vi "Periodic Tasks.vi"(8 "error in":errorcluster) -> ()   [LabVIEW 2016]
doc: "This VI runs in parallel to other tasks. It can contain as many user-defined periodic loops as you need. These can carry out PID or other sorts of timed response."
uses:
  <vilib>/Rock Robotics/WPI/Solenoid/WPI_SolenoidValue.ctl
  <vilib>/Rock Robotics/WPI/DriverStation/WPI_DriverStationRobotMode2.ctl
  <vilib>/Rock Robotics/WPI/Utilities/WPI_GetSetVariantRefNum.vi
  Robot Global Data.vi
  <vilib>/Rock Robotics/WPI/Solenoid/WPI_SolenoidSetEnum.vi
  Added Files/Apple Gyro/Apple Pi Gyro Library.lvlib
panel:
  out "Robot Centric?":bool
  in  "Turn":dbl=0.7 format="%#_13g"
  in  "Harvest Spd":dbl=0.9 format="%#_13g"
  out "Output":bool
  out "Intake":bool
  in  "Output":i32=6
  in  "Intake":i32=4
  out "Gyro Yaw Out 2":dbl format="%#_13g"
  in  "Rot Pt Y":dbl format="%#_13g"
  in  "Rot Pt X":dbl format="%#_13g"
  in  "Robot Centric":i32
  in  "Field Centric":i32
  in  "Y Axis":i32=1
  in  "Drive wait":u32=25
  out "Drive Loop Speed":u32=245
  in  "Slow Drive Speed %":dbl=0.65
  in  "OP wait":u32=25
  out "Op Loop Speed":u32=138
  out "Joystick Loop Speed":u32=39
  in  "Joystick wait":u32=25
  out "Reset Offsets":bool
  out "Vision Lineup":bool
  out "Driver 2 POV":i16=-1
  out "Climb":bool
  in  "Reset Offsets":i32=7
  in  "Lineup":i32
  in  "Drive Slow":i32=1
  in  "Gyro Reset":i32=2
  in  "Climb":i32=1
  in  "Max Climb Speed":dbl=-1.0
  # "Left Driver 1"
  # "Right Driver 2"
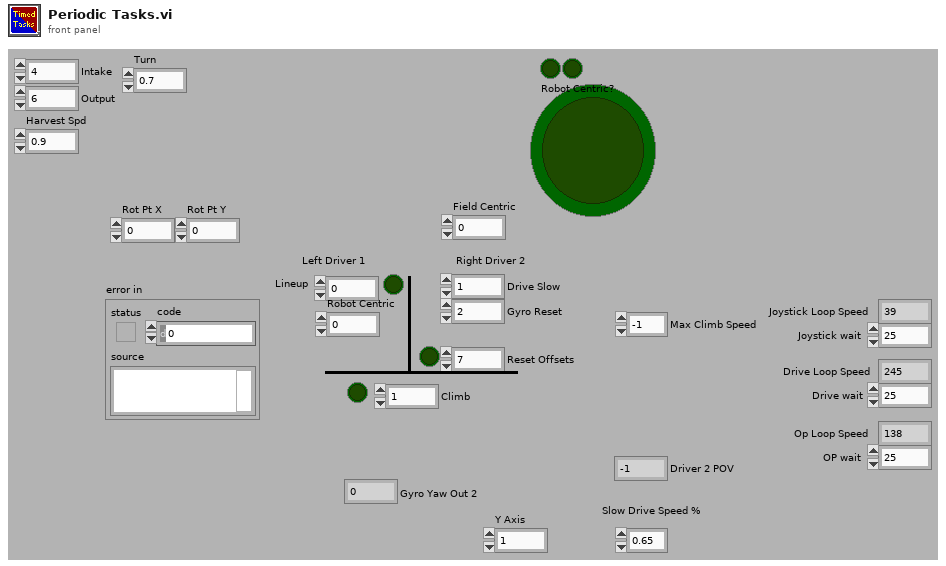
[diagram p1: front panel]
types:
  T1 = typedef "WPI_JoystickDevRef.ctl" = cluster{"Device":T2}
  T2 = typedef "WPI_JoystickDeviceEnum.ctl" = enum16{"USB 0", "USB 1", "USB 2", "USB 3", "USB 4", "USB 5"}
  T3 = typedef "WPI_DriverStationRobotMode2.ctl" = enum16{"Autonomous Disabled", "Autonomous Enabled", "Teleop Disabled", "Teleop Enabled", "Disconnected", "Finish", "Test Disabled", "Test Enabled", "Emergency Stopped"}
  T4 = typedef "WPI_MotorControlDeviceRef.ctl" = cluster{"DeviceStatus":errorcluster, "Type":T5, "PWM":cluster{"PWM Channel":T6, "DeadBand":T7}, "CAN":cluster{"Device Number":u8, "SetOutput VI Ref":variant, "GetOutput VI Ref":variant, "Enable VI Ref":variant, "Disable VI Ref":variant, "Data":variant}, "Invert":bool}
  T5 = typedef "WPI_MotorControlType.ctl" = enum16{"PWM", "CAN"}
  T6 = typedef "FPGA_DIOPWMChannel.ctl" = enum8{"PWM 0", "PWM 1", "PWM 2", "PWM 3", "PWM 4", "PWM 5", "PWM 6", "PWM 7", "PWM 8", "PWM 9", "PWM MXP 0", "PWM MXP 1", "PWM MXP 2", "PWM MXP 3", "PWM MXP 4", "PWM MXP 5", "PWM MXP 6", "PWM MXP 7", "PWM MXP 8", "PWM MXP 9", "Invalid"}
  T7 = typedef "WPI_PWMDeadband.ctl" = cluster{"Name":string, "maxPositivePwm":i32, "minPositivePwm":i32, "centerPwm":i32, "maxNegativePwm":i32, "minNegativePwm":i32, "angularRange":u16}
  T8 = typedef "WPI_SolenoidDevRef.ctl" = cluster{"DevStatus":errorcluster, "Pneumatics Control Module":u8, "Forward Solenoid Channel":T9, "Reverse Solenoid Channel":T9}
  T9 = typedef "WPI_SolenoidChannel.ctl" = enum8{"Solenoid 0", "Solenoid 1", "Solenoid 2", "Solenoid 3", "Solenoid 4", "Solenoid 5", "Solenoid 6", "Solenoid 7", "Invalid"}
  T10 = typedef "WPI_SolenoidValue.ctl" = enum16{"Off", "On", "Forward", "Reverse"}
  T11 = typedef "WPI_CompressorDevRef.ctl" = cluster{"DevStatus":errorcluster, "Pneumatics Control Module":u8}
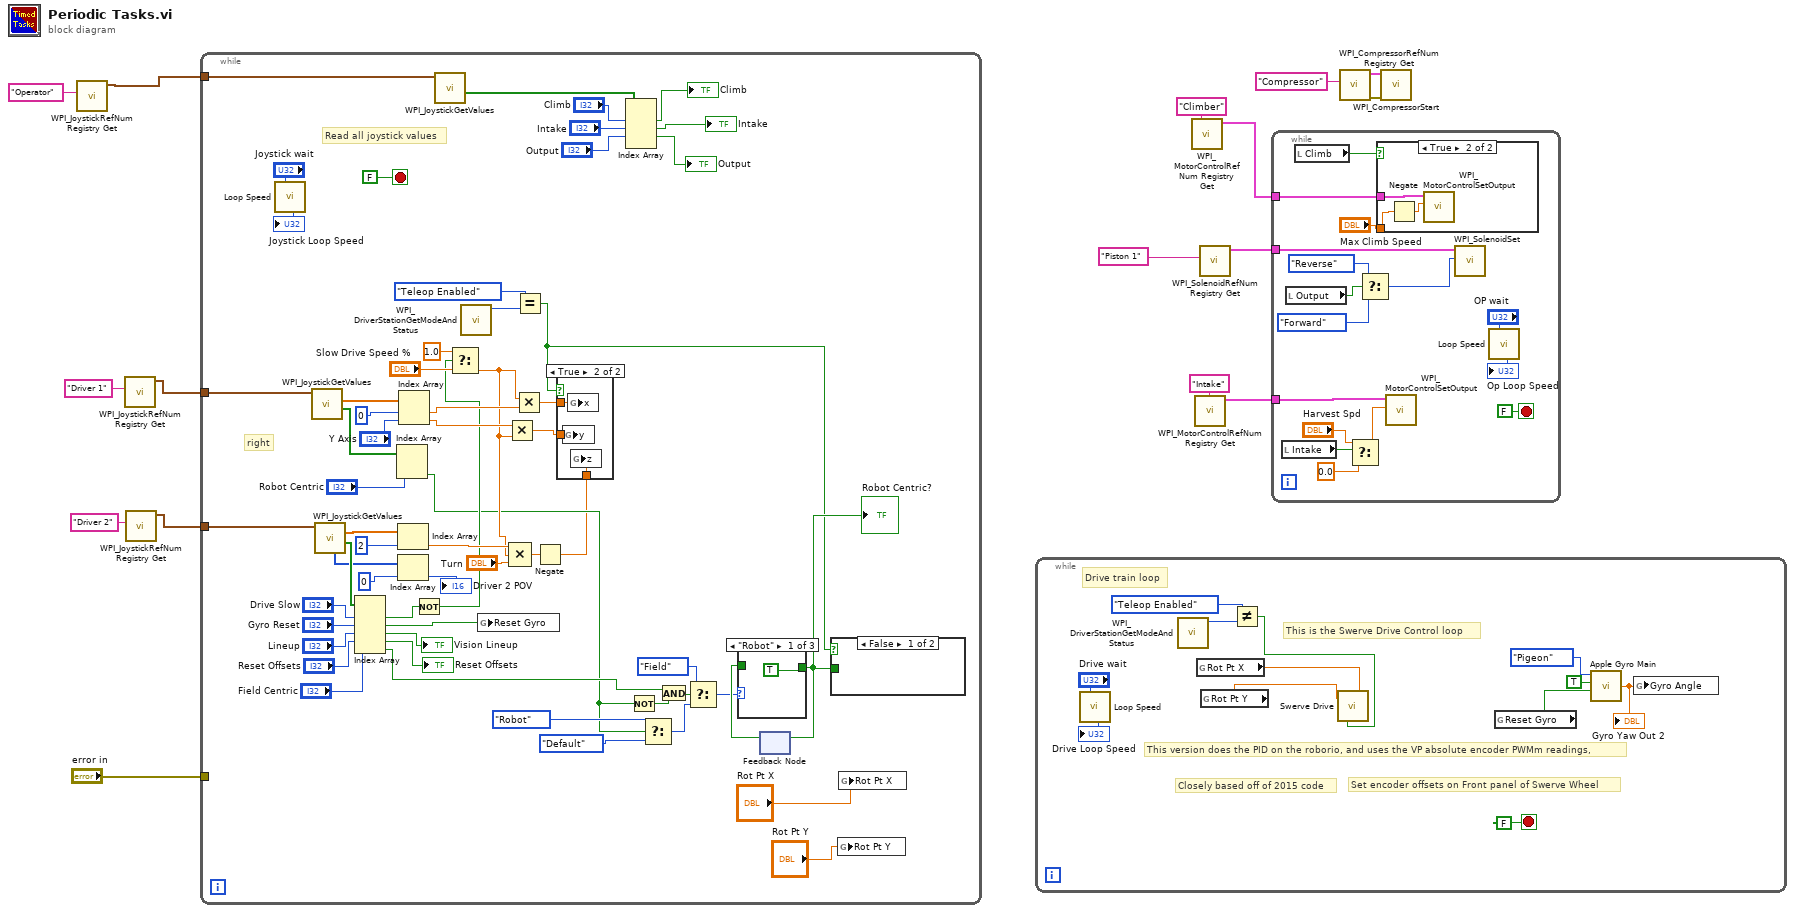
[diagram p0: block diagram]
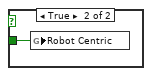
[diagram p2: hidden frame]
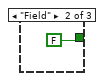
[diagram p4: hidden frame]
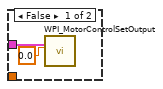
[diagram p6: hidden frame]
diagram:
  n1 = call <vilib>:"WPI_JoystickRefNum Registry Get.vi"("refnum name"="Operator") -> ("JoystickDevRef"=w11:T1)  [unwired: 9 in, 1 out]
  n2 = call <vilib>:"WPI_JoystickRefNum Registry Get.vi"("refnum name"="Driver 1") -> ("JoystickDevRef"=w10:T1)  [unwired: 9 in, 1 out]
  n3 = call <vilib>:"WPI_JoystickRefNum Registry Get.vi"("refnum name"="Driver 2") -> ("JoystickDevRef"=w9:T1)  [unwired: 9 in, 1 out]
  n4 = while {
    tunnel: w11 -> [w45]
    tunnel: w10 -> [w44]
    tunnel: w9 -> [w43]
    tunnel: "error in" -> [_]
    stop <- FALSE stop-if-true
    # "Read all joystick values"
    # "right"
    n5 = call "Loop Speed.vi"("milliseconds to wait"="Joystick wait") -> ("Loop Speed"=→"Joystick Loop Speed":u32)
    n6 = call <vilib>:"WPI_JoystickGetValues.vi"("JoystickDevRef"=w44) -> ("Buttons"=w64:bool[], "Axes"=w73:dbl[])  [unwired: 6 in, 3 out]
    n7 = call <vilib>:"WPI_JoystickGetValues.vi"("JoystickDevRef"=w43) -> ("Buttons"=w71:bool[], "Axes"=w72:dbl[], "POVs"=w65:i16[])  [unwired: 6 in, 2 out]
    n8 = Index Array(array=w71, index #1="Drive Slow", index #2="Gyro Reset", index #3="Lineup", index #4="Reset Offsets", index #5="Field Centric") -> (element #1=w49:bool, element #2=w48:bool, element #3=→"Vision Lineup":bool, element #4=→"Reset Offsets":bool, element #5=w31:bool)
    n9 = Index Array(array=w64, index #2="Robot Centric") -> (element #2=w29:bool)  [unwired: 1 in, 1 out]
    n10 = Index Array(array=w72, index=2) -> (element=w61:dbl)
    n11 = Index Array(array=w65, index=0) -> (element=→"Driver 2 POV":i16)
    n12 = Index Array(array=w73, index #1=0 ("index"), index #2="Y Axis") -> (element #1=w63:dbl, element #2=w62:dbl)
    n13 = Not(x=w49) -> (.not. x?=w47:bool)
    n14 = call <vilib>:"WPI_JoystickGetValues.vi"("JoystickDevRef"=w45) -> ("Buttons"=w76:bool[])  [unwired: 6 in, 4 out]
    n15 = Select(t=1.0, s=w47, f="Slow Drive Speed %") -> (s? t:f=w51:dbl)
    n16 = call <vilib>:"WPI_DriverStationGetModeAndStatus.vi"() -> ("Robot Mode"=w19:T3)  [unwired: 10 in, 1 out]
    n17 = global write "Robot Global Data.vi" "Reset Gyro"(w48) -> ()
    n18 = Multiply(x=w62, y=w51) -> (x*y=w53:dbl)
    n19 = Compound Arithmetic op=MULTIPLY(w61, w51, "Turn") -> (w42:dbl)
    n20 = Multiply(x=w51, y=w63) -> (x*y=w52:dbl)
    n21 = Equal?(x=WPI_DriverStationRobotMode2."Teleop Enabled", y=w19) -> (x = y?=w17:bool)
    n22 = Negate(x=w42) -> (-x=w20:dbl)
    n23 = case shown="True" w17 {
      tunnel: w53 -> [_ w81]
      tunnel: w52 -> [_ w80]
      tunnel: w20 -> [_ w79]
      frame False {
      }
      frame True {
        n24 = global write "Robot Global Data.vi" "y"(w81) -> ()
        n25 = global write "Robot Global Data.vi" "x"(w80) -> ()
        n26 = global write "Robot Global Data.vi" "z"(w79) -> ()
      }
    }
    n27 = Index Array(array=w76, index #1="Climb", index #2="Intake", index #3="Output") -> (element #1=→"Climb":bool, element #2=→"Intake":bool, element #3=→"Output":bool)  [unwired: 1 in, 1 out]
    n28 = Not(x=w29) -> (.not. x?=w39:bool)
    n29 = Select(t=enum16{"Field", "Robot", "Default"}."Robot", s=w29, f=enum16{"Field", "Robot", "Default"}."Default") -> (s? t:f=w35:enum16{"Field", "Robot", "Default"})
    n30 = And(x=w31, y=w39) -> (x .and. y?=w34:bool)
    n31 = Select(t=enum16{"Field", "Robot", "Default"}."Field", s=w34, f=w35) -> (s? t:f=w36:enum16{"Field", "Robot", "Default"})
    n32 = feedback #1() -> (w40:bool)  [unwired: 1 in]
    n33 = case shown="\"Robot\"" w36 {
      tunnel: [TRUE FALSE w84] -> w41
      tunnel: w40 -> [_ _ w84]
      frame "Robot" {
      }
      frame "Field" {
      }
      frame Default {
      }
    }
    "Robot Centric?" <- w41
    n34 = feedback-in #1(w41) -> ()
    n35 = case shown="False" w17 {
      tunnel: w41 -> [_ w78]
      frame False {
      }
      frame True {
        n36 = global write "Robot Global Data.vi" "Robot Centric"(w78) -> ()
      }
    }
    n37 = global write "Robot Global Data.vi" "Rot Pt Y"("Rot Pt Y") -> ()
    n38 = global write "Robot Global Data.vi" "Rot Pt X"("Rot Pt X") -> ()
  }
  n39 = while {
    stop <- FALSE stop-if-true
    # "Set encoder offsets on Front panel of Swerve Wheel"
    # "Closely based off of 2015 code"
    # "This version does the PID on the roborio, and uses the VP absolute encoder PWMm readings,"
    # "This is the Swerve Drive Control loop"
    # "Drive train loop"
    n40 = call "Loop Speed.vi"("milliseconds to wait"="Drive wait") -> ("Loop Speed"=→"Drive Loop Speed":u32)
    n41 = call <vilib>:"WPI_DriverStationGetModeAndStatus.vi"() -> ("Robot Mode"=w91:T3)  [unwired: 10 in, 1 out]
    n42 = global read "Robot Global Data.vi" "Rot Pt X"() -> (w92:dbl)
    n43 = global read "Robot Global Data.vi" "Rot Pt Y"() -> (w93:dbl)
    n44 = Not Equal?(x=WPI_DriverStationRobotMode2."Teleop Enabled", y=w91) -> (x != y?=w89:bool)
    n45 = call "Swerve Drive.vi"("Rot. Point Y"=w93, "Rot. Point X"=w92, "Auto Controls"=w89) -> ()  [unwired: 13 in]
    n46 = global read "Robot Global Data.vi" "Reset Gyro"() -> (w87:bool)
    n47 = call "Apple Gyro Main.vi"("Reset All"=w87, "Override NT?"=TRUE, "Gyro Select (Overide)"=enum16{"IMU", "SPI", "Analog", "Navx", "Pigeon"}."Pigeon") -> ("Gyro Yaw Out"=w86:dbl)  [unwired: 1 in]
    "Gyro Yaw Out 2" <- w86
    n48 = global write "Robot Global Data.vi" "Gyro Angle"(w86) -> ()
  }
  n49 = call <vilib>:"WPI_MotorControlRefNum Registry Get.vi"("refnum name"="Climber") -> ("MotorControlDevRef"=w15:T4)  [unwired: 9 in, 1 out]
  n50 = call <vilib>:"WPI_MotorControlRefNum Registry Get.vi"("refnum name"="Intake") -> ("MotorControlDevRef"=w1:T4)  [unwired: 9 in, 1 out]
  n51 = call <vilib>:"WPI_SolenoidRefNum Registry Get.vi"("refnum name"="Piston 1") -> ("SolenoidDevRef"=w4:T8)  [unwired: 9 in, 1 out]
  n52 = while {
    tunnel: w15 -> [w107]
    tunnel: w4 -> [w104]
    tunnel: w1 -> [w103]
    stop <- FALSE stop-if-true
    n53 = local read "Intake"() -> (w99:bool)
    n54 = local read "Output"() -> (w101:bool)
    n55 = local read "Climb"() -> (w112:bool)
    n56 = Select(t="Harvest Spd", s=w99, f=0.0) -> (s? t:f=w100:dbl)
    n57 = Select(t=WPI_SolenoidValue."Reverse" ("Value"), s=w101, f=WPI_SolenoidValue."Forward" ("Value")) -> (s? t:f=w102:T10)
    n58 = case shown="True" w112 {
      tunnel: w107 -> [w113 w117]
      tunnel: "Max Climb Speed" -> [_ w115]
      frame False {
        n59 = call <vilib>:"WPI_MotorControlSetOutput.vi"("Output"=0.0, "MotorControlDevRef"=w113) -> ()  [unwired: 7 in, 3 out]
      }
      frame True {
        n60 = Negate(x=w115) -> (-x=w116:dbl)
        n61 = call <vilib>:"WPI_MotorControlSetOutput.vi"("Output"=w116, "MotorControlDevRef"=w117) -> ()  [unwired: 7 in, 3 out]
      }
    }
    n62 = call <vilib>:"WPI_MotorControlSetOutput.vi"("Output"=w100, "MotorControlDevRef"=w103) -> ()  [unwired: 7 in, 3 out]
    n63 = call-poly <vilib>:"WPI_SolenoidSet.vi"("Value"=w102, "SolenoidDevRef"=w104) -> ()  [unwired: 8 in, 2 out]
    n64 = call "Loop Speed.vi"("milliseconds to wait"="OP wait") -> ("Loop Speed"=→"Op Loop Speed":u32)
  }
  n65 = call <vilib>:"WPI_CompressorRefNum Registry Get.vi"("refnum name"="Compressor") -> ("error out"=w5:errorcluster, "CompressorDevRef"=w7:T11)  [unwired: 9 in]
  n66 = call <vilib>:"WPI_CompressorStart.vi"("error in (no error)"=w5, "CompressorDevRef"=w7) -> ()  [unwired: 8 in, 2 out]
